vi "Front Panel2.vi"() -> ()   [LabVIEW 2020]
uses:
  GL_SetpointDispl.vi
  GL_TempUnits.vi
  GL_Pgain.vi
  GL_Ireset.vi
  GL_Drate.vi
  GL_heaterdisplay.vi
  GL_HeaterOn.vi
  GL_SamplerateDispl.vi
  GL_TempDspl.vi
  GL_MHeaterDisplay.vi
panel:
  in  "STOP":bool=TRUE
  out "D":dbl min=0.0 max=100.0 step=0.01 format="%.2f"
  out "I":dbl min=0.0 max=100.0 step=0.01 format="%.2f"
  out "P":dbl min=0.0 max=100.0 step=0.01 format="%.2f"
  out "MANUAL HEATER DISPLAY":dbl(slide) caption="AMP" min=0.0 max=5.0 scale=0.0..5.0
  out "HEATER ON":bool
  out "Array":bool[](array[boolean])
  in  "SETUP / ADJUST":bool
  out "SAMPLE RATE (sec)":dbl=1.0 min=0.0 max=600.0 step=0.01 format="%.3f"
  out "SET POINT":dbl min=0.0 max=450.0 step=0.0001 format="%.4f"
  out "unit":enum16{"K", "Ohms", "C", "F"}(ring)
  out "TEMPERATURE\nDisplay":dbl format="%.3f"
  # "e"
  # "e"
  # "TEMPERATURE \nREMOTE TEMPERATURE CONTROLLER"
  # "TEMPERATURE \nREMOTE TEMPERATURE CONTROLLER"
  # "SET  POINT"
  # "SET  POINT"
  # "SAMPLE RATE (sec)"
  # "remote manual heater control\nnot functioning"
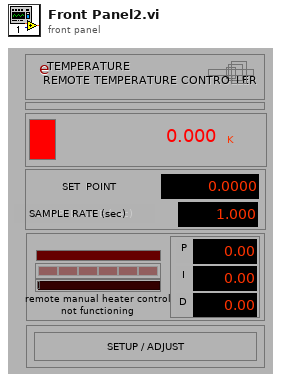
[diagram p1: front panel]
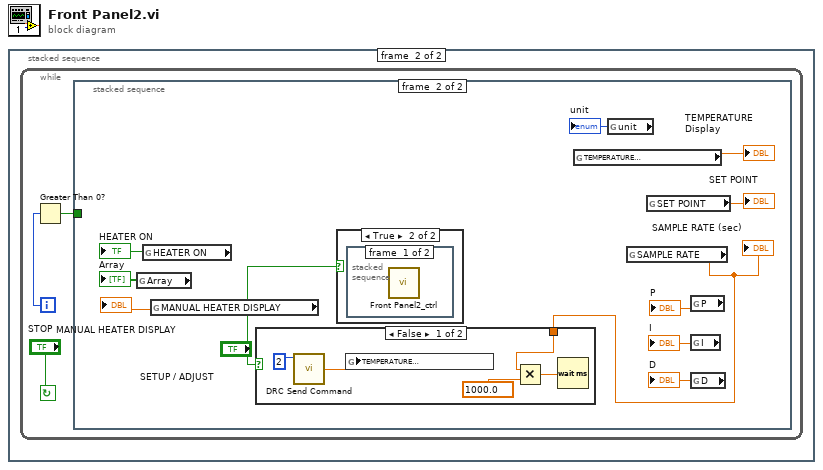
[diagram p0: block diagram]
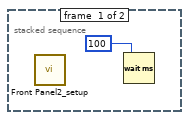
[diagram p2: hidden frame]
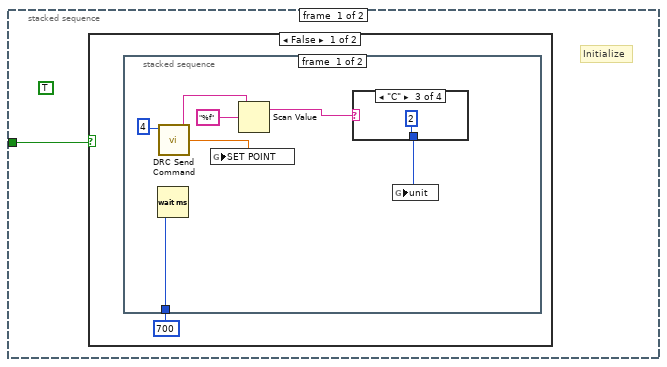
[diagram p3: hidden frame]
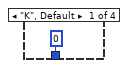
[diagram p4: hidden frame]
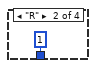
[diagram p5: hidden frame]
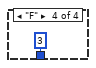
[diagram p6: hidden frame]
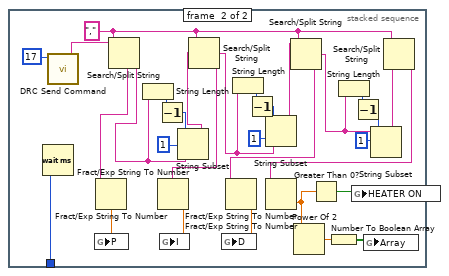
[diagram p7: hidden frame]
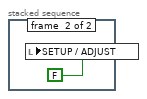
[diagram p10: hidden frame]
diagram:
  n1 = stacked-sequence {
    frame #0 {
      n2 = call "Front Panel2_setup.vi"() -> ()  [unwired: 3 in, 1 out]
      n3 = Wait (ms)(milliseconds to wait=100) -> ()  [unwired: 1 out]
    }
    frame #1 {
      n4 = while {
        i -> [w3]
        stop <- "STOP" continue-if-true
        n5 = Greater Than 0?(x=w3) -> (x > 0?=w2:bool)
        n6 = stacked-sequence {
          tunnel: w2 -> [w5 _]
          frame #0 {
            (unwired) TRUE
            # "Initialize"
            n7 = case shown="False" w5 {
              frame False {
                n8 = stacked-sequence {
                  tunnel: 700 -> [w12 w46]
                  frame #0 {
                    n9 = Wait (ms)(milliseconds to wait=w12) -> ()  [unwired: 1 out]
                    n10 = call "DRC Send Command.vi"("Command"=4) -> ("Output"=w8:dbl, "Response"=w11:string)  [unwired: 3 in, 1 out]
                    n11 = global write "GL_SetpointDispl.vi" "SET POINT"(w8) -> ()
                    n12 = Scan Value(string=w11, format string="%f") -> (output string=w7:string)  [unwired: 1 in, 1 out]
                    n13 = case shown="\"C\"" w7 {
                      tunnel: [0 1 2 3] -> w9
                      frame "K", Default {
                      }
                      frame "R" {
                      }
                      frame "C" {
                      }
                      frame "F" {
                      }
                    }
                    n14 = global write "GL_TempUnits.vi" "unit"(w9) -> ()
                  }
                  frame #1 {
                    w45 = ","
                    n15 = Wait (ms)(milliseconds to wait=w46) -> ()  [unwired: 1 out]
                    n16 = call "DRC Send Command.vi"("Command"=17) -> ("Response"=w36:string)  [unwired: 3 in, 2 out]
                    n17 = Search/Split String(string=w36, search string/char (-)=w45) -> (substring before match=w44:string, match + rest of string=w22:string)  [unwired: 1 in, 1 out]
                    n18 = Fract/Exp String To Number(string=w44) -> (number=w43:dbl)  [unwired: 3 in, 1 out]
                    n19 = global write "GL_Pgain.vi" "P"(w43) -> ()
                    n20 = String Length(string=w22) -> (length=w24:i32)
                    n21 = Decrement(x=w24) -> (x-1=w23:i32)
                    n22 = String Subset(string=w22, offset (0)=1, length (rest)=w23) -> (substring=w34:string)
                    n23 = Search/Split String(string=w34, search string/char (-)=w45) -> (substring before match=w21:string, match + rest of string=w25:string)  [unwired: 1 in, 1 out]
                    n24 = Fract/Exp String To Number(string=w21) -> (number=w42:dbl)  [unwired: 3 in, 1 out]
                    n25 = global write "GL_Ireset.vi" "I"(w42) -> ()
                    n26 = String Length(string=w25) -> (length=w27:i32)
                    n27 = Decrement(x=w27) -> (x-1=w26:i32)
                    n28 = String Subset(string=w25, offset (0)=1, length (rest)=w26) -> (substring=w32:string)
                    n29 = Search/Split String(string=w32, search string/char (-)=w45) -> (substring before match=w31:string, match + rest of string=w28:string)  [unwired: 1 in, 1 out]
                    n30 = Fract/Exp String To Number(string=w31) -> (number=w41:dbl)  [unwired: 3 in, 1 out]
                    n31 = global write "GL_Drate.vi" "D"(w41) -> ()
                    n32 = String Length(string=w28) -> (length=w30:i32)
                    n33 = Decrement(x=w30) -> (x-1=w29:i32)
                    n34 = String Subset(string=w28, offset (0)=1, length (rest)=w29) -> (substring=w37:string)
                    n35 = Search/Split String(string=w37, search string/char (-)=w45) -> (substring before match=w18:string)  [unwired: 1 in, 2 out]
                    n36 = Fract/Exp String To Number(string=w18) -> (number=w19:dbl)  [unwired: 3 in, 1 out]
                    n37 = Power Of 2(x=w19) -> (2^x=w20:dbl)
                    n38 = Greater Than 0?(x=w19) -> (x > 0?=w40:bool)
                    n39 = Number To Boolean Array(number=w20) -> (Boolean array=w39:bool[])
                    n40 = global write "GL_HeaterOn.vi" "HEATER ON"(w40) -> ()
                    n41 = global write "GL_heaterdisplay.vi" "Array"(w39) -> ()
                  }
                }
              }
              frame True {
              }
            }
          }
          frame #1 {
            n42 = global read "GL_heaterdisplay.vi" "Array"() -> (→"Array":bool[])
            n43 = global read "GL_HeaterOn.vi" "HEATER ON"() -> (→"HEATER ON":bool)
            n44 = global read "GL_MHeaterDisplay.vi" "MANUAL HEATER DISPLAY"() -> (→"MANUAL HEATER DISPLAY":dbl)
            n45 = case shown="True" "SETUP / ADJUST" {
              frame False {
              }
              frame True {
                n46 = stacked-sequence {
                  frame #0 {
                    n47 = call "Front Panel2_ctrl.vi"() -> ()  [unwired: 2 in, 1 out]
                  }
                  frame #1 {
                    n48 = local write "SETUP / ADJUST"(FALSE) -> ()
                  }
                }
              }
            }
            n49 = global read "GL_TempDspl.vi" "TEMPERATURE\nDisplay"() -> (→"TEMPERATURE\nDisplay":dbl)
            n50 = global read "GL_TempUnits.vi" "unit"() -> (→"unit":enum16{"K", "Ohms", "C", "F"})
            n51 = global read "GL_SamplerateDispl.vi" "SAMPLE RATE"() -> (w48:dbl)
            "SAMPLE RATE (sec)" <- w48
            n52 = case shown="False" "SETUP / ADJUST" {
              tunnel: w48 -> [w60 _]
              frame False {
                n53 = call "DRC Send Command.vi"("Command"=2) -> ("Output"=w64:dbl)  [unwired: 3 in, 2 out]
                n54 = global write "GL_TempDspl.vi" "TEMPERATURE\nDisplay"(w64) -> ()
                n55 = Multiply(x=w60, y=1000.0) -> (x*y=w62:dbl)
                n56 = Wait (ms)(milliseconds to wait=w62) -> ()  [unwired: 1 out]
              }
              frame True {
              }
            }
            n57 = global read "GL_SetpointDispl.vi" "SET POINT"() -> (→"SET POINT":dbl)
            n58 = global read "GL_Pgain.vi" "P"() -> (→"P":dbl)
            n59 = global read "GL_Ireset.vi" "I"() -> (→"I":dbl)
            n60 = global read "GL_Drate.vi" "D"() -> (→"D":dbl)
          }
        }
      }
    }
  }
